vi "Closed loop test.vi"() -> ()   [LabVIEW 2014]
uses:
  <vilib>/Platform/TimedLoop/XDataNode/timing_clust.ctl
  <vilib>/Platform/TimedLoop/XDataNode/nitl_modes.ctl
  <vilib>/Platform/TimedLoop/XDataNode/wakeup.ctl
  <vilib>/rvi/FXPMathLib/basic elements/FxpIntAccumulator/subVIs/nifxpmath_IntAccumulator_SimConfig.ctl
  <vilib>/rvi/FXPMathLib/FxpSqrt/subVIs/nifxpmath_Sqrt_SimConfig.ctl
  <vilib>/fxp/LVFixedPointOverflowPolicyTypeDef.ctl
  <vilib>/rvi/eio/common/nirviEmuTemplateMethod_errors.vi
  <vilib>/rvi/Emulation/niFpgaSctlEmulationGetInTimedLoop.vi
  <vilib>/rvi/Emulation/niFpgaEmulationReportErrorSimple.vi
  <vilib>/rvi/Emulation/niFpgaGetClockAttributes.vi
  <vilib>/rvi/Emulation/niFpgaCriticalErrorInLSC.vi
  <vilib>/rvi/Analysis/common/codeGenErrors/XNode/niFpgaXNodeCodeGenErrorHandle.vi
  <vilib>/rvi/FXPMathLib/basic elements/FxpIntAccumulator/simVIs/DllFxpIntAccumulator_sub.vi
  <vilib>/rvi/FXPMathLib/FxpSqrt/simVIs/DllSqrtTemp_sub.vi
  <vilib>/rvi/Memory/Memory_Emulation/nirvimemoryFastEmulation.vi
  <vilib>/rvi/Memory/Memory_Emulation/nirvimemoryEmulation.vi
  <vilib>/rvi/Emulation/niFpgaEmulationIsFPGAContextNoSignature.vi
  <vilib>/rvi/DataTransferAndStorage/Container/Common/niFpgaContainerGetUniqueNameForEmu.vi
  <vilib>/rvi/Emulation/niFpgaProcessEmulError.vi
  <vilib>/rvi/errors/nirviReportUnexpectedCaseInternalError (U32).vi
  <vilib>/eio/EIOMethodNode/EIOMethodNode.xnode
  <vilib>/Platform/TimedLoop/XDataNode/XDataNode.xnode
  <vilib>/rvi/Analysis/measure/dc-rms/XNode/niFpgaDC-RMS.xnode
  <vilib>/rvi/FXPMathLib/FxpMul/XNode/nifxpmath_Multiplier.xnode
  <vilib>/rvi/FXPMathLib/basic elements/FxpIntAccumulator/XNode/nifxpmath_IntAccumulator.xnode
  <vilib>/rvi/FXPMathLib/FxpSqrt/XNode/nifxpmath_Sqrt.xnode
  <vilib>/rvi/DataTransferAndStorage/Container/XNode/niFpgaContainer.xnode
  <vilib>/Platform/TimedLoop/XDataNode/XDNodeRunTimeDep.lvlib
  <vilib>/rvi/FXPMathLib/sim/FxpSim.dll
panel:
  out "RMS":fxp<+,12,12>
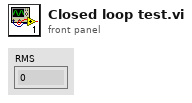
[diagram p1: front panel]
types:
  T1 = typedef "XDNodeRunTimeDep.lvlib/timing_clust.ctl" = cluster{"Expected End [f-1]":u64, "Actual End [f-1]":u64, "Finished Late? [f-1]":bool, "Expected End [i-1]":u64, "Actual End [i-1]":u64, "Finished Late? [i-1]":bool, "Expected Start [i]":u64, "Actual Start [i]":u64, "Expected Start [f]":u64, "Actual Start [f]":u64, "Source Name":string, "Structure Name":string, "Period":i64, "Deadline":i64, "Offset":i64, "Start":i64, "Priority":i32, "Timeout":i32, "Mode":T2, "Wakeup Reason":T3, "Error":errorcluster, "Source Type":string, "Secondary Source Type":string, "Global End Time":u64, "Global Start Time":u64, "Frame Duration":u64, "Iteration Duration":u64, "Assigned CPU":i32, "I/O Scan Engine Mode":u32}
  T2 = typedef "XDNodeRunTimeDep.lvlib/nitl_modes.ctl" = enum32{"No Change", "Process missed periods, maintain original phase", "Discard missed periods, maintain original phase", "Process missed periods, ignore original phase", "Discard missed periods, ignore original phase"}
  T3 = typedef "XDNodeRunTimeDep.lvlib/wakeup.ctl" = enum32{"Normal", "Aborted", "Asynchronous wakeup", "Timing source error", "Timed loop error", "Timeout"}
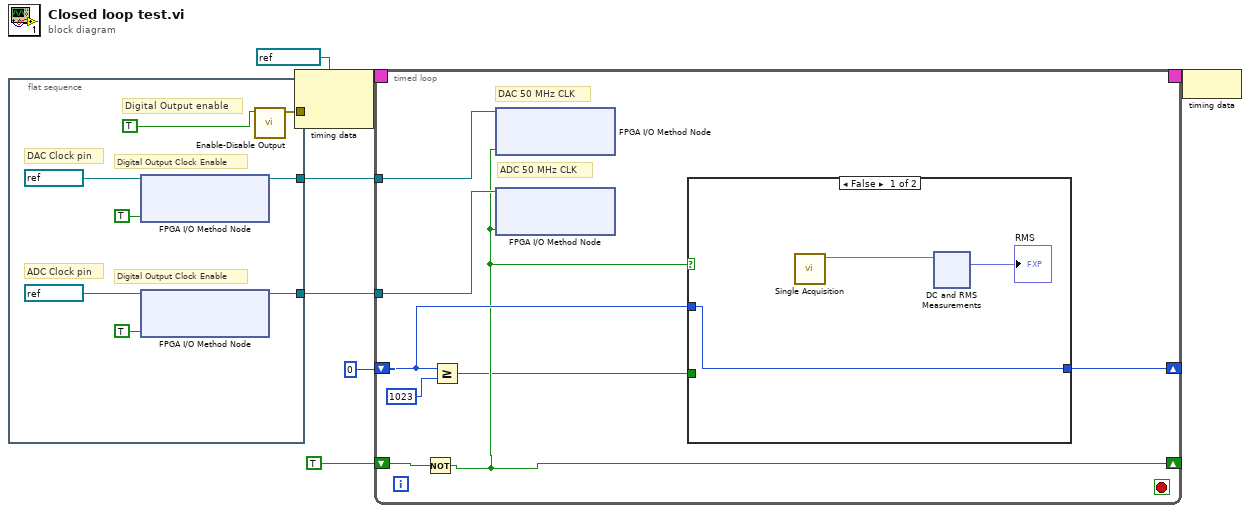
[diagram p0: block diagram]
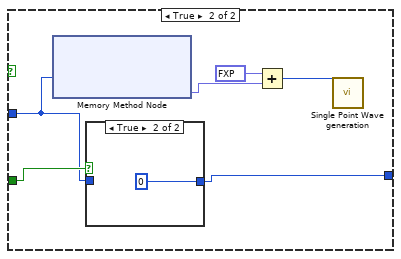
[diagram p2: hidden frame]
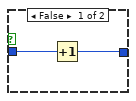
[diagram p3: hidden frame]
diagram:
  n1 = flat-sequence {
    tunnel: [w14] -> w5
    tunnel: [w12] -> w3
    tunnel: [w9] -> w4
    frame #0 {
      # "Digital Output Clock Enable"
      # "DAC Clock pin"
      # "Digital Output Clock Enable"
      # "Digital Output enable"
      # "ADC Clock pin"
      n2 = xnode "FPGA I/O Method Node"("FPGA I/O In"=refnum<k21> "DIO16", "Enable"=TRUE) -> ("FPGA I/O Out"=w9:refnum<k21>)
      n3 = xnode "FPGA I/O Method Node"("FPGA I/O In"=refnum<k21> "DIO17", "Enable"=TRUE) -> ("FPGA I/O Out"=w14:refnum<k21>)
      n4 = call "Enable-Disable Output.vi"("Enable"=TRUE) -> ("error out"=w12:errorcluster)  [unwired: 10 in]
    }
  }
  n5 = node-c288(refnum<k21> "2.5MHz" ("Source Name"), w3) -> (w8:T1)
  n6 = timed-loop {
    timing: w8 -> [_]
    timing-out: [_] -> w7
    tunnel: w5 -> [w24]
    tunnel: w4 -> [w23]
    shift-right: [w19] -> _
    shift-left: TRUE ("Enable") -> [w20]
    shift-right: [w17] -> _
    shift-left: u32 0 -> [w21]
    stop <- _ stop-if-true
    # "DAC 50 MHz CLK"
    # "ADC 50 MHz CLK"
    n7 = Not(x=w20) -> (.not. x?=w19:bool)
    n8 = Greater Or Equal?(x=w21, y=u32 1023) -> (x >= y?=w18:bool)
    n9 = xnode "FPGA I/O Method Node"("FPGA I/O In"=w23, "Data"=w19) -> ()  [unwired: 1 out]
    n10 = xnode "FPGA I/O Method Node"("FPGA I/O In"=w24, "Data"=w19) -> ()  [unwired: 1 out]
    n11 = case shown="False" w19 {
      tunnel: w21 -> [w25 w152]
      tunnel: w18 -> [_ w154]
      tunnel: [w25 w153] -> w17
      frame False {
        n12 = call "Single Acquisition.vi"() -> ("Out"=w27:fxp<+/-,12,12>)  [unwired: 11 in]
        n13 = xnode "DC and RMS Measurements"("input data"=w27) -> ("RMS"=→"RMS":fxp<+,12,12>)  [unwired: 3 in, 2 out]
      }
      frame True {
        n14 = xnode ("Memory Method Node")("Address"=w152) -> ("Data"=w151:fxp<+/-,12,12>)  [unwired: 1 in, 1 out]
        n15 = case shown="True" w154 {
          tunnel: [w155 u32 0] -> w153
          tunnel: w152 -> [w156 _]
          frame False {
            n16 = Increment(x=w156) -> (x+1=w155:u32)
          }
          frame True {
          }
        }
        n17 = Add(x=fxp<+/-,12,12> 2047.0, y=w151) -> (x+y=w149:u16)
        n18 = call "Single Point Wave generation.vi"("Data To Write"=w149) -> ()  [unwired: 10 in, 1 out]
      }
    }
  }
  n19 = node-c288(w7) -> ()
